vi "ClusterTest.vi"(11 "error in":errorcluster) -> (15 "error out":errorcluster)   [LabVIEW 2016]
uses:
  <vilib>/addons/_JKI Toolkits/Caraya/classes/Assert/Assert Equal Value and Type_Variant.vi
  <vilib>/addons/_JKI Toolkits/Caraya/classes/Assert/Assert.lvclass
  <vilib>/addons/_JKI Toolkits/Caraya/classes/Test/Test.lvclass
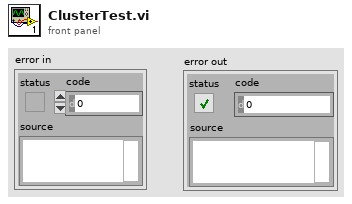
[diagram p1: front panel]
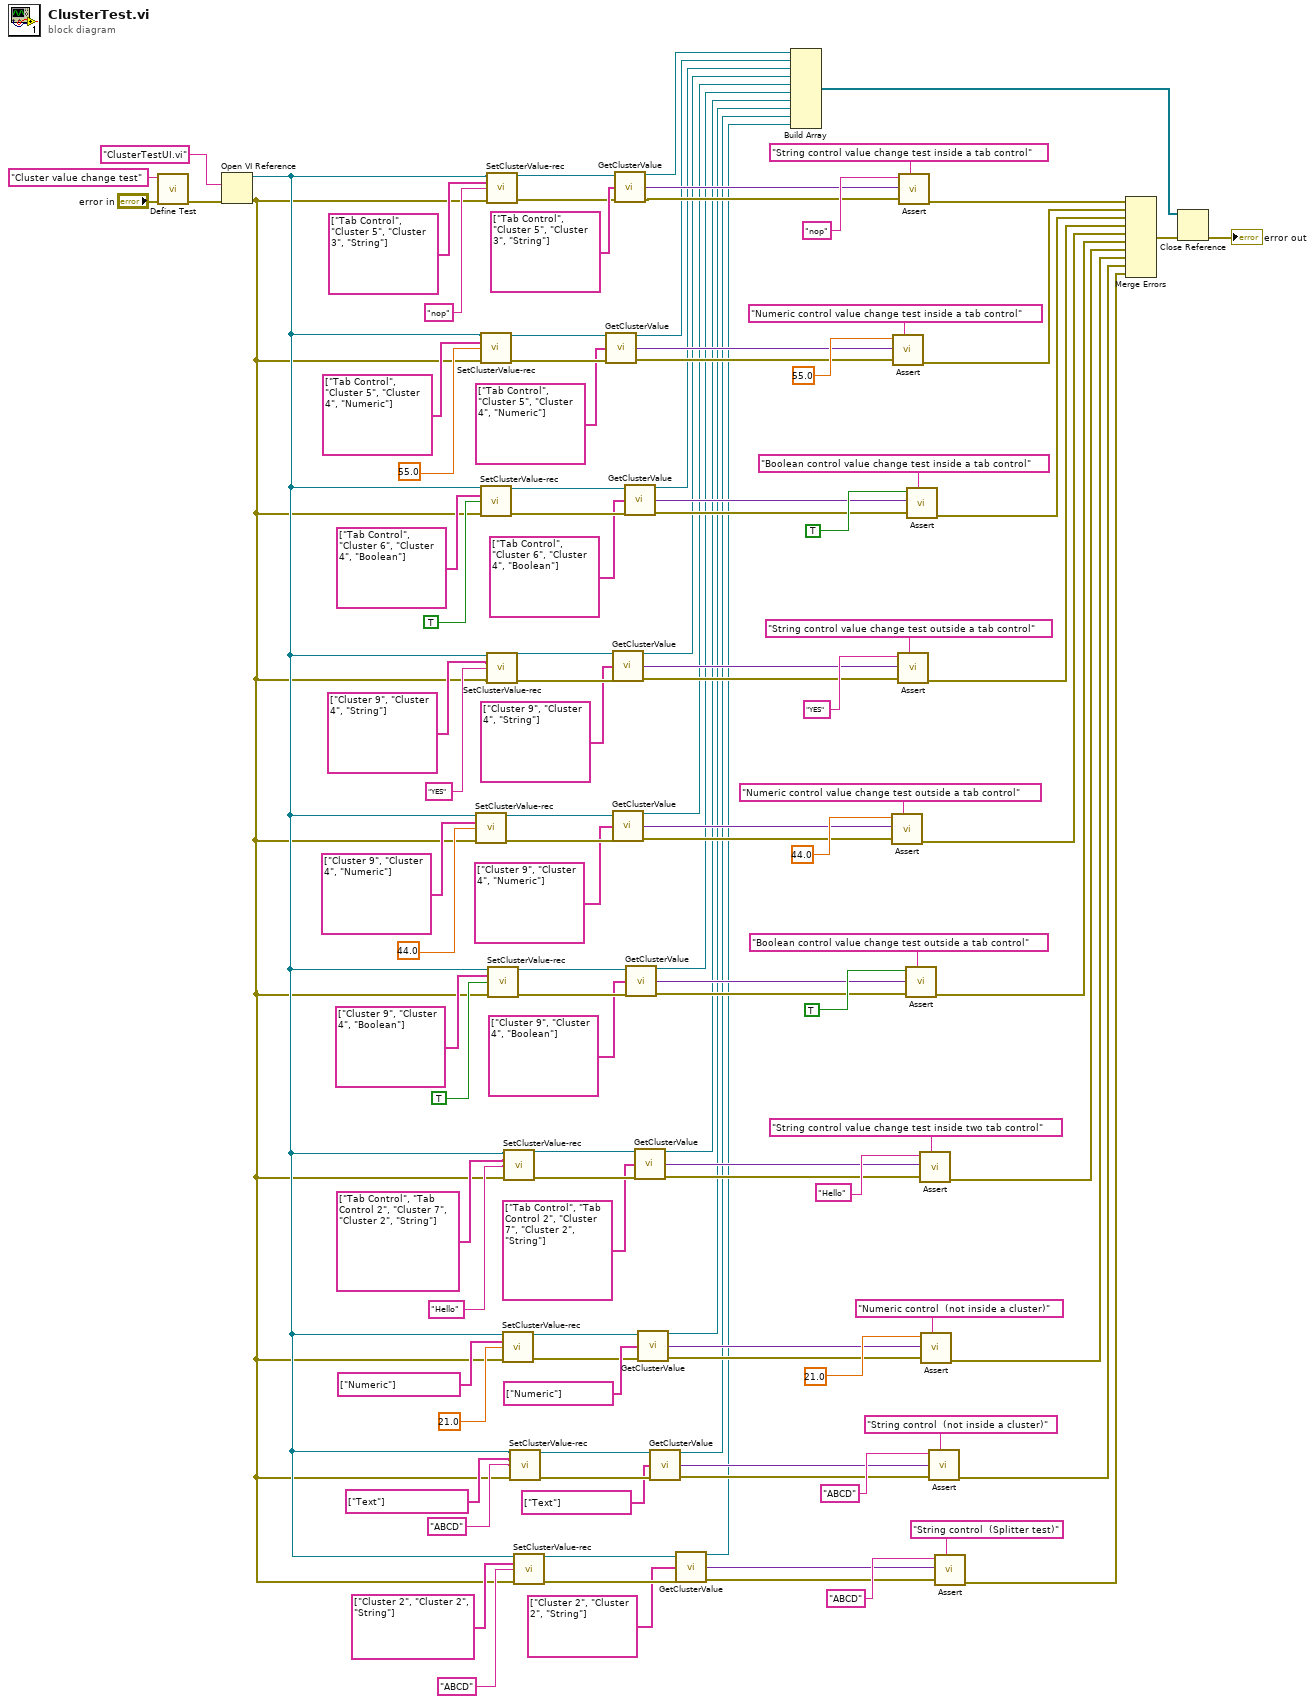
[diagram p0: block diagram]
diagram:
  n1 = call <vilib>:"Define Test.vi"("error in (no error)"="error in", "Label (VI Title)"="Cluster value change test") -> ("error out"=w115:errorcluster)  [unwired: 9 in]
  n2 = Open VI Reference(vi path="ClusterTestUI.vi", error in (no error)=w115) -> (vi reference=w64:refnum<vi>, error out=w61:errorcluster)  [unwired: 4 in]
  n3 = call "SetClusterValue-rec.vi"("VI Reference"=w64, "Array"=string[] ["Cluster 9", "Cluster 4", "Numeric"], "Control Value"=44.0, "error in"=w61) -> ("VI Reference out"=w32:refnum<vi>, "error out"=w33:errorcluster)  [unwired: 10 in]
  n4 = call "SetClusterValue-rec.vi"("VI Reference"=w64, "Array"=string[] ["Tab Control", "Cluster 5", "Cluster 4", "Numeric"], "Control Value"=55.0, "error in"=w61) -> ("VI Reference out"=w49:refnum<vi>, "error out"=w54:errorcluster)  [unwired: 10 in]
  n5 = call "SetClusterValue-rec.vi"("VI Reference"=w64, "Array"=string[] ["Tab Control", "Cluster 6", "Cluster 4", "Boolean"], "Control Value"=TRUE, "error in"=w61) -> ("VI Reference out"=w44:refnum<vi>, "error out"=w45:errorcluster)  [unwired: 10 in]
  n6 = call "SetClusterValue-rec.vi"("VI Reference"=w64, "Array"=string[] ["Tab Control", "Cluster 5", "Cluster 3", "String"], "Control Value"="nop" ("Control Name"), "error in"=w61) -> ("VI Reference out"=w57:refnum<vi>, "error out"=w55:errorcluster)  [unwired: 10 in]
  n7 = call "SetClusterValue-rec.vi"("VI Reference"=w64, "Array"=string[] ["Cluster 9", "Cluster 4", "String"], "Control Value"="YES" ("Control Name"), "error in"=w61) -> ("VI Reference out"=w38:refnum<vi>, "error out"=w39:errorcluster)  [unwired: 10 in]
  n8 = call "SetClusterValue-rec.vi"("VI Reference"=w64, "Array"=string[] ["Cluster 9", "Cluster 4", "Boolean"], "Control Value"=TRUE, "error in"=w61) -> ("VI Reference out"=w26:refnum<vi>, "error out"=w27:errorcluster)  [unwired: 10 in]
  n9 = call "SetClusterValue-rec.vi"("VI Reference"=w64, "Array"=string[] ["Numeric"], "Control Value"=21.0, "error in"=w61) -> ("VI Reference out"=w13:refnum<vi>, "error out"=w14:errorcluster)  [unwired: 10 in]
  n10 = call "SetClusterValue-rec.vi"("VI Reference"=w64, "Array"=string[] ["Tab Control", "Tab Control 2", "Cluster 7", "Cluster 2", "String"], "Control Value"="Hello", "error in"=w61) -> ("VI Reference out"=w20:refnum<vi>, "error out"=w21:errorcluster)  [unwired: 10 in]
  n11 = call "SetClusterValue-rec.vi"("VI Reference"=w64, "Array"=string[] ["Text"], "Control Value"="ABCD", "error in"=w61) -> ("VI Reference out"=w8:refnum<vi>, "error out"=w9:errorcluster)  [unwired: 10 in]
  n12 = call "SetClusterValue-rec.vi"("VI Reference"=w64, "Array"=string[] ["Cluster 2", "Cluster 2", "String"], "Control Value"="ABCD", "error in"=w61) -> ("VI Reference out"=w2:refnum<vi>, "error out"=w3:errorcluster)  [unwired: 10 in]
  n13 = call "GetClusterValue.vi"("VI Reference"=w49, "Array"=string[] ["Tab Control", "Cluster 5", "Cluster 4", "Numeric"], "error in"=w54) -> ("VI Reference out"=w53:refnum<vi>, "Value"=w52:variant, "error out"=w51:errorcluster)  [unwired: 10 in]
  n14 = call "GetClusterValue.vi"("VI Reference"=w38, "Array"=string[] ["Cluster 9", "Cluster 4", "String"], "error in"=w39) -> ("VI Reference out"=w42:refnum<vi>, "Value"=w41:variant, "error out"=w40:errorcluster)  [unwired: 10 in]
  n15 = call "GetClusterValue.vi"("VI Reference"=w32, "Array"=string[] ["Cluster 9", "Cluster 4", "Numeric"], "error in"=w33) -> ("VI Reference out"=w36:refnum<vi>, "Value"=w35:variant, "error out"=w34:errorcluster)  [unwired: 10 in]
  n16 = call "GetClusterValue.vi"("VI Reference"=w57, "Array"=string[] ["Tab Control", "Cluster 5", "Cluster 3", "String"], "error in"=w55) -> ("VI Reference out"=w60:refnum<vi>, "Value"=w59:variant, "error out"=w58:errorcluster)  [unwired: 10 in]
  n17 = call "GetClusterValue.vi"("VI Reference"=w44, "Array"=string[] ["Tab Control", "Cluster 6", "Cluster 4", "Boolean"], "error in"=w45) -> ("VI Reference out"=w48:refnum<vi>, "Value"=w47:variant, "error out"=w46:errorcluster)  [unwired: 10 in]
  n18 = call "GetClusterValue.vi"("VI Reference"=w26, "Array"=string[] ["Cluster 9", "Cluster 4", "Boolean"], "error in"=w27) -> ("VI Reference out"=w30:refnum<vi>, "Value"=w29:variant, "error out"=w28:errorcluster)  [unwired: 10 in]
  n19 = call "GetClusterValue.vi"("VI Reference"=w20, "Array"=string[] ["Tab Control", "Tab Control 2", "Cluster 7", "Cluster 2", "String"], "error in"=w21) -> ("VI Reference out"=w24:refnum<vi>, "Value"=w23:variant, "error out"=w22:errorcluster)  [unwired: 10 in]
  n20 = call "GetClusterValue.vi"("VI Reference"=w13, "Array"=string[] ["Numeric"], "error in"=w14) -> ("VI Reference out"=w18:refnum<vi>, "Value"=w17:variant, "error out"=w16:errorcluster)  [unwired: 10 in]
  n21 = call "GetClusterValue.vi"("VI Reference"=w8, "Array"=string[] ["Text"], "error in"=w9) -> ("VI Reference out"=w12:refnum<vi>, "Value"=w11:variant, "error out"=w10:errorcluster)  [unwired: 10 in]
  n22 = call "GetClusterValue.vi"("VI Reference"=w2, "Array"=string[] ["Cluster 2", "Cluster 2", "String"], "error in"=w3) -> ("VI Reference out"=w6:refnum<vi>, "Value"=w5:variant, "error out"=w4:errorcluster)  [unwired: 10 in]
  n23 = Build Array(w60, w53, w48, w42, w36, w30, w24, w18, w12, w6) -> (w113:refnum<vi>[])
  n24 = call-poly <vilib>:"Assert.vi"("Label"="Numeric control value change test outside a tab control", "error in (no error)"=w34, "Y"=w35, "X"=44.0) -> ("error out"=w96:errorcluster)  [unwired: 7 in]
  n25 = call-poly <vilib>:"Assert.vi"("Label"="Numeric control value change test inside a tab control", "error in (no error)"=w51, "Y"=w52, "X"=55.0) -> ("error out"=w111:errorcluster)  [unwired: 7 in]
  n26 = call-poly <vilib>:"Assert.vi"("Label"="String control value change test outside a tab control", "error in (no error)"=w40, "Y"=w41, "X"="YES" ("Control Name")) -> ("error out"=w97:errorcluster)  [unwired: 7 in]
  n27 = call-poly <vilib>:"Assert.vi"("Label"="String control value change test inside a tab control", "error in (no error)"=w58, "Y"=w59, "X"="nop" ("Control Name")) -> ("error out"=w110:errorcluster)  [unwired: 7 in]
  n28 = call-poly <vilib>:"Assert.vi"("Label"="Boolean control value change test outside a tab control", "error in (no error)"=w28, "Y"=w29, "X"=TRUE) -> ("error out"=w95:errorcluster)  [unwired: 7 in]
  n29 = call-poly <vilib>:"Assert.vi"("Label"="Boolean control value change test inside a tab control", "error in (no error)"=w46, "Y"=w47, "X"=TRUE) -> ("error out"=w106:errorcluster)  [unwired: 7 in]
  n30 = call-poly <vilib>:"Assert.vi"("Label"="String control value change test inside two tab control", "error in (no error)"=w22, "Y"=w23, "X"="Hello") -> ("error out"=w94:errorcluster)  [unwired: 7 in]
  n31 = call-poly <vilib>:"Assert.vi"("Label"="Numeric control  (not inside a cluster)", "error in (no error)"=w16, "Y"=w17, "X"=21.0) -> ("error out"=w89:errorcluster)  [unwired: 7 in]
  n32 = call-poly <vilib>:"Assert.vi"("Label"="String control  (not inside a cluster)", "error in (no error)"=w10, "Y"=w11, "X"="ABCD") -> ("error out"=w87:errorcluster)  [unwired: 7 in]
  n33 = call-poly <vilib>:"Assert.vi"("Label"="String control  (Splitter test)", "error in (no error)"=w4, "Y"=w5, "X"="ABCD") -> ("error out"=w83:errorcluster)  [unwired: 7 in]
  n34 = Merge Errors(w110, w111, w106, w97, w96, w95, w94, w89, w87, w83) -> (w109:errorcluster)
  n35 = Close Reference(reference=w113, error in (no error)=w109) -> (error out=→"error out":errorcluster)
